vi "~CSC_CableTension2JointForce.vi"(8 "error in (no error)":errorcluster, 10 "CableTension":dbl[](array[numeric]), 11 "C-Alex in":refnum<class "CableSerialChain.lvclass">) -> (0 "error out":errorcluster, 3 "C-Alex out":refnum<class "CableSerialChain.lvclass">)   [LabVIEW 2015, in "CableSerialChain.lvclass"]
uses:
  CableSerialChain.lvclass
  <vilib>/Analysis/BLAS.llb/dnrm2 - Vector 2-Norm (DBL).vi
  <vilib>/Analysis/NI_AALBLAS.lvlib
  <vilib>/Analysis/NI_AALPro.lvlib
panel:
  out "CableLength":dbl[](array[numeric])
  out "Joint Force Knee":dbl[](array[numeric]) format="%#.6f"
  out "Joint Force Hip":dbl[](array[numeric]) format="%#.6f"
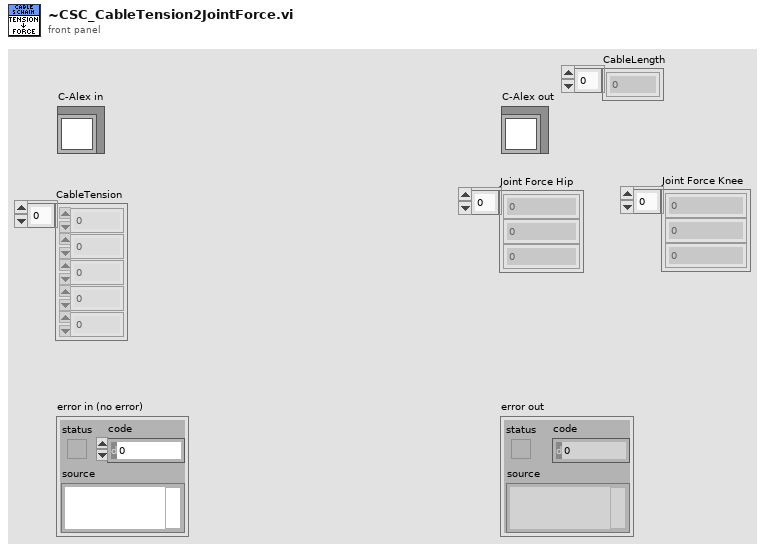
[diagram p1: front panel]
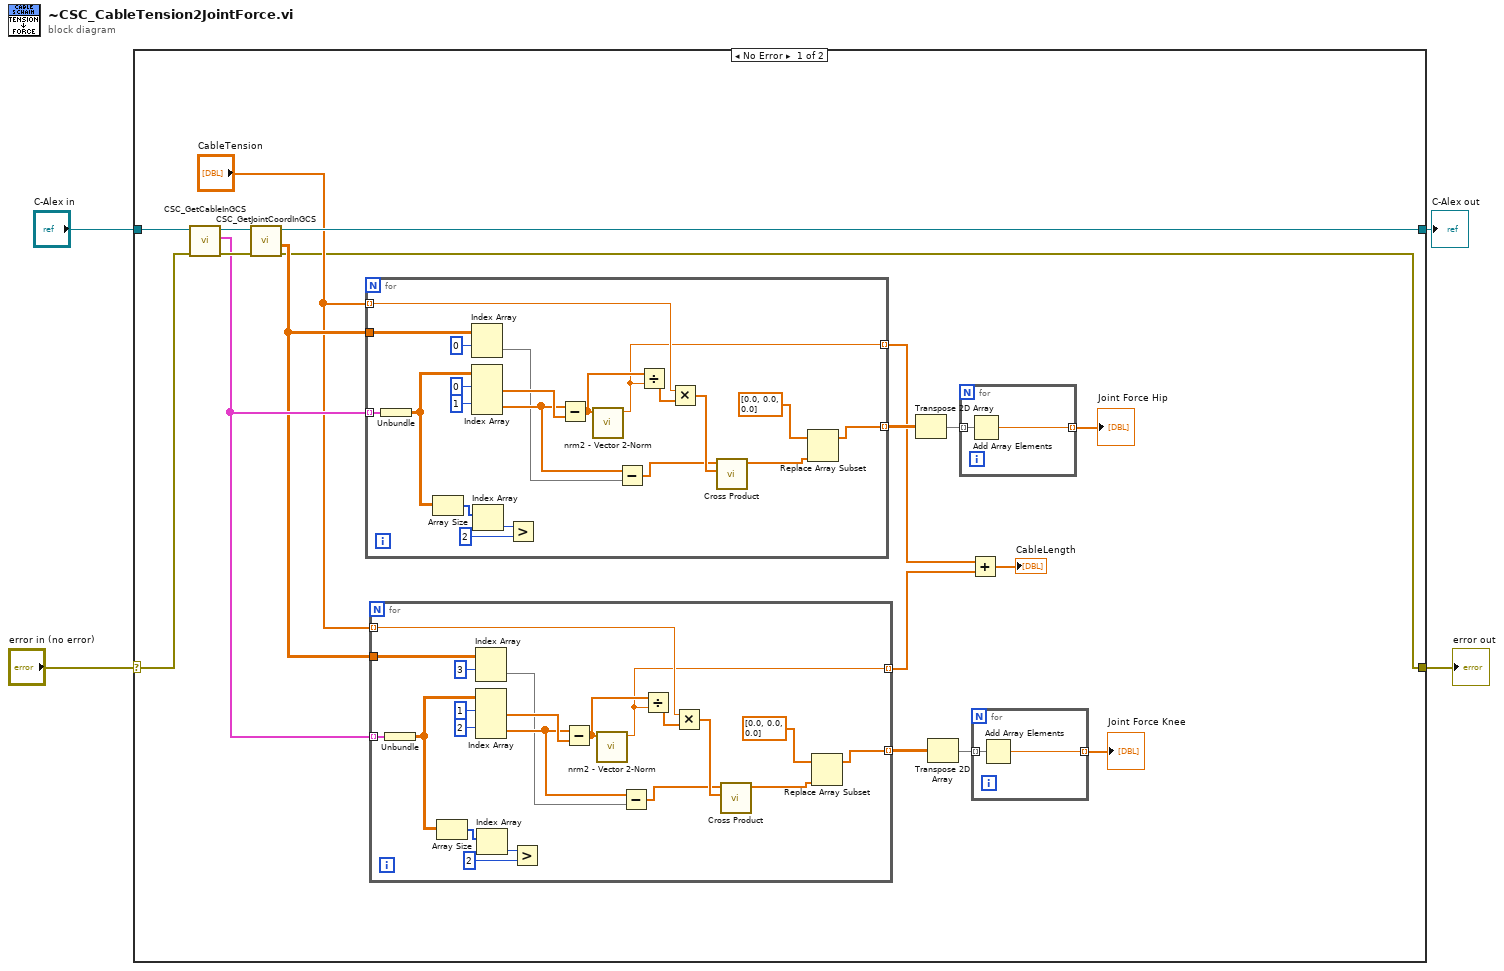
[diagram p0: block diagram]
diagram:
  n1 = case shown="No Error" "error in (no error)" {
    selector: "error in (no error)" -> [w17 w69]
    tunnel: [w5 w69] -> w3
    tunnel: [w15 w70] -> w1
    tunnel: "C-Alex in" -> [w22 w70]
    frame No Error {
      n2 = call "CSC_GetCableInGCS.vi"("error in (no error)"=w17, "C-Alex in"=w22) -> ("error out"=w14:errorcluster, "Cables Points"=w13:cluster{"PointInGCS":dbl[][]}[], "C-Alex out"=w16:refnum<class "CableSerialChain.lvclass">)  [unwired: 7 in]
      n3 = call "CSC_GetJointCoordInGCS.vi"("error in (no error)"=w14, "C-Alex in"=w16) -> ("error out"=w5:errorcluster, "Jcoord & End Eff in GCS"=w12:dbl[][], "C-Alex out"=w15:refnum<class "CableSerialChain.lvclass">)  [unwired: 6 in, 1 out]
      n4 = for {
        tunnel: w13 -> [w43] mode=indexing
        tunnel: "CableTension" -> [w39] mode=indexing
        tunnel: [w24] -> w10 mode=indexing
        tunnel: w12 -> [w35]
        tunnel: [w23] -> w9 mode=indexing
        n5 = Unbundle(w43) -> ("PointInGCS"=w30:dbl[][])
        n6 = Array Size(array=w30) -> (size(s)=w29:i32[])
        n7 = Index Array(array=w35, index (row)=0) -> (element=w31:dbl[])  [unwired: 1 in]
        n8 = Index Array(array=w30, index (row) #1=0 ("index (row)"), index (row) #2=1 ("index (row)")) -> (element #1=w41:dbl[], element #2=w33:dbl[])  [unwired: 2 in]
        n9 = Index Array(array=w29) -> (element=w28:i32)  [unwired: 1 in]
        n10 = Greater?(x=w28, y=2) -> ()  [unwired: 1 out]
        n11 = Subtract(x=w33, y=w41) -> (x-y=w40:dbl[])
        n12 = call-poly <vilib>:"nrm2 - Vector 2-Norm.vi"("x"=w40) -> ("dnrm2"=w23:dbl)  [unwired: 9 in, 1 out]
        n13 = Subtract(x=w33, y=w31) -> (x-y=w32:dbl[])
        n14 = Divide(x=w40, y=w23) -> (x/y=w38:dbl[])
        n15 = Multiply(x=w39, y=w38) -> (x*y=w37:dbl[])
        n16 = call <vilib>:"Cross Product.vi"("B Vector"=w37, "A Vector"=w32) -> ("Cross Product"=w26:dbl[])  [unwired: 8 in, 1 out]
        n17 = Replace Array Subset(array=dbl[] [0.0, 0.0, 0.0] ("JointSpeed"), new element=w26) -> (w24:dbl[])  [unwired: 1 in]
      }
      n18 = for {
        tunnel: w13 -> [w66] mode=indexing
        tunnel: "CableTension" -> [w62] mode=indexing
        tunnel: [w47] -> w20 mode=indexing
        tunnel: w12 -> [w58]
        tunnel: [w46] -> w21 mode=indexing
        n19 = Unbundle(w66) -> ("PointInGCS"=w53:dbl[][])
        n20 = Array Size(array=w53) -> (size(s)=w52:i32[])
        n21 = Index Array(array=w58, index (row)=3) -> (element=w54:dbl[])  [unwired: 1 in]
        n22 = Index Array(array=w53, index (row) #1=1 ("index (row)"), index (row) #2=2 ("index (row)")) -> (element #1=w64:dbl[], element #2=w56:dbl[])  [unwired: 2 in]
        n23 = Index Array(array=w52) -> (element=w51:i32)  [unwired: 1 in]
        n24 = Greater?(x=w51, y=2) -> ()  [unwired: 1 out]
        n25 = Subtract(x=w56, y=w64) -> (x-y=w63:dbl[])
        n26 = call-poly <vilib>:"nrm2 - Vector 2-Norm.vi"("x"=w63) -> ("dnrm2"=w46:dbl)  [unwired: 9 in, 1 out]
        n27 = Subtract(x=w56, y=w54) -> (x-y=w55:dbl[])
        n28 = Divide(x=w63, y=w46) -> (x/y=w61:dbl[])
        n29 = Multiply(x=w62, y=w61) -> (x*y=w60:dbl[])
        n30 = call <vilib>:"Cross Product.vi"("B Vector"=w60, "A Vector"=w55) -> ("Cross Product"=w49:dbl[])  [unwired: 8 in, 1 out]
        n31 = Replace Array Subset(array=dbl[] [0.0, 0.0, 0.0] ("JointSpeed"), new element=w49) -> (w47:dbl[])  [unwired: 1 in]
      }
      n32 = Transpose 2D Array(2D array=w10) -> (transposed array=w18:dbl[][])
      n33 = Transpose 2D Array(2D array=w20) -> (transposed array=w19:dbl[][])
      n34 = for {
        tunnel: w18 -> [w68] mode=indexing
        tunnel: [w67] -> w8 mode=indexing
        n35 = Add Array Elements(numeric array=w68) -> (sum=w67:dbl)
      }
      "Joint Force Hip" <- w8
      n36 = Add(x=w9, y=w21) -> (x+y=→"CableLength":dbl[])
      n37 = for {
        tunnel: w19 -> [w45] mode=indexing
        tunnel: [w44] -> w7 mode=indexing
        n38 = Add Array Elements(numeric array=w45) -> (sum=w44:dbl)
      }
      "Joint Force Knee" <- w7
    }
    frame Error {
    }
  }
  "error out" <- w3
  "C-Alex out" <- w1
